vi "Read Minor Frame Period.vi"(8 "error in":errorcluster, 11 "port":T1 format="%.0x") -> (0 "error out":errorcluster, 2 "minor frame period (us)":i32, 3 "port out":T1 format="%.0x")   [LabVIEW 2020, in "AIM MIL-STD-1553 Scripting.lvlib"]
uses:
  AIM MIL-STD-1553 Scripting.lvlib
  <vilib>/NI VeriStand/Custom Device API/Custom Device Item Ref.ctl
  Constants.vi
  <vilib>/NI VeriStand/Custom Device API/Get Item Property (Double).vi
  <vilib>/NI VeriStand/Custom Device API/Custom Device API.lvlib
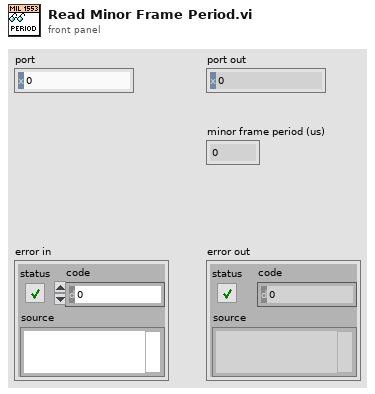
[diagram p1: front panel]
types:
  T1 = typedef "Custom Device API.lvlib/Custom Device Item Ref.ctl" = u64
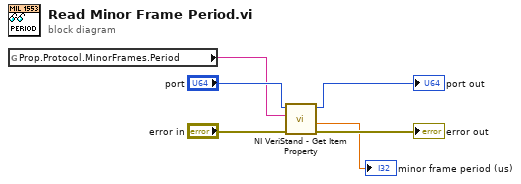
[diagram p0: block diagram]
diagram:
  n1 = global read "Constants.vi" "Prop.Protocol.MinorFrames.Period"() -> (w5:string)
  n2 = call-poly <vilib>:"NI VeriStand - Get Item Property.vi"("error in (no error)"="error in", "Property Name"=w5, "Item Ref in"="port") -> ("error out"=→"error out":errorcluster, "Value"=→"minor frame period (us)":dbl, "Item Ref out"=→"port out":T1)  [unwired: 5 in, 1 out]
